vi "Read Txt File as Lines LV2016.vi"(8 "error in":errorcluster, 10 "Lines to Read":i32, 11 "file path (use dialog)":path) -> (0 "error out":errorcluster, 3 "Lines":string[](array[string]))   [LabVIEW 2016]
doc: "This Function is designed to read in a text file and retunr an array of string with each line of the text file. \n\nFor comments or questions about this code please look at the community example page below.\nhttp://decibel.ni.com/content/docs/DOC-10662"
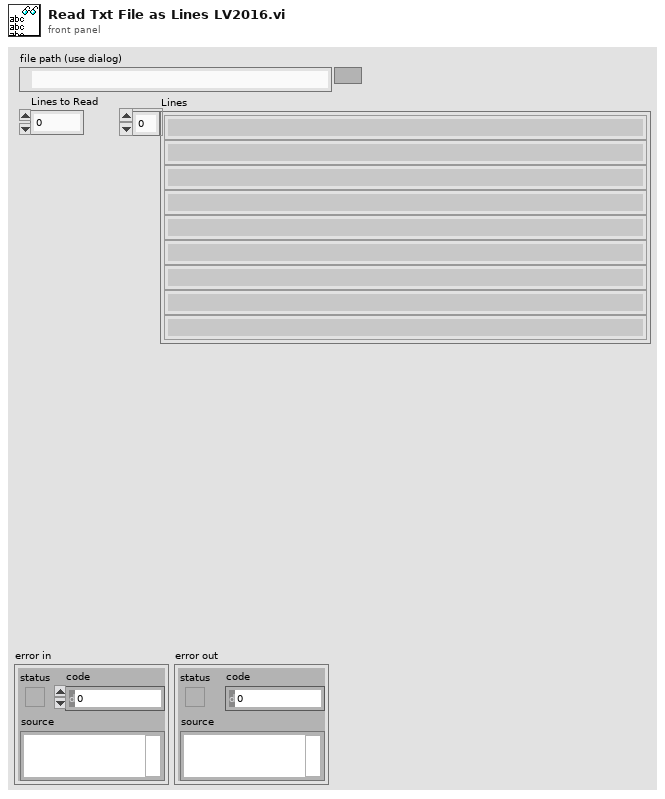
[diagram p1: front panel]
types:
  T1 = enum16{"open", "replace", "create", "open or create", "replace or create", "replace or create with confirmation"}
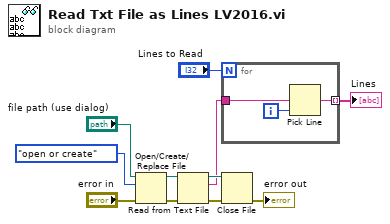
[diagram p0: block diagram]
diagram:
  n1 = Open/Create/Replace File(file path (use dialog)="file path (use dialog)", error in="error in", operation (0:open)=T1."open or create") -> (refnum out=w11:refnum<file>, error out=w10:errorcluster)  [unwired: 3 in, 1 out]
  n2 = Read from Text File(file (use dialog)=w11, error in=w10) -> (refnum out=w6:refnum<file>, text=w4:string, error out=w7:errorcluster)  [unwired: 2 in, 1 out]
  n3 = for {
    N: "Lines to Read" -> [_]
    tunnel: w4 -> [w13]
    tunnel: [w12] -> w3 mode=indexing
    i -> [w14]
    n4 = Pick Line(multi-line string=w13, line index=w14) -> (output string=w12:string)  [unwired: 1 in]
  }
  "Lines" <- w3
  n5 = Close File(refnum=w6, error in=w7) -> (error out=→"error out":errorcluster)  [unwired: 1 out]
